vi "Teleop.vi"(10 "Match Info":T1={"Autonomous Elapsed Seconds"=0.0, "TeleOp Elapsed Seconds"=0.0, "Disabled Elapsed Seconds"=0.0, "Visited Autonomous"=FALSE, "Visited TeleOp"=FALSE, "Visited Disabled"=FALSE, "Autonomous Settings"={"Autonomous Style"=enum."Independent", "VI Refnum"=refnum}}, 11 "Call Context":T2) -> ()   [LabVIEW 2019]
doc: "This VI is called for each enabled TeleOp packet received from the DS. It is typically used to read from joysticks and other inputs and update I/O or setpoints for timed control loops. It should complete and return within 20 milliseconds or risk missing DS packets."
uses:
  <vilib>/Rock Robotics/WPI/DriverStation/WPI_DriverStationDerivedRobotMode.ctl
  <vilib>/Rock Robotics/WPI/DriverStation/WPI_DriverStationMatch Info.ctl
  Drive/Implementation/Drive Globals.vi
  <vilib>/Rock Robotics/Network Tables/NT Write Numeric Array.vi
  <vilib>/Rock Robotics/Network Tables/NT Write Boolean Array.vi
panel:
  out "Roller Velocity":dbl
  out "Left LIft Applied Voltage":dbl
  out "Right Drive Velocity":dbl
  out "Left Drive Velocity":dbl
  out "Right LIft Velocity":dbl
  out "Left LIft Velocity":dbl
  out "LeftStopped":bool
  out "RightStopped":bool
  out "Bottom Limit  Pressed":bool
  out "ArmSpeed":dbl
  out "ArmDirection":bool
  out "ArmPosition":dbl
  out "RightDriveSpeed":dbl
  out "RightDriveDirection":bool
  out "RightDriveDistance":dbl
  out "Left Drive Speed":dbl
  out "LeftDriveDirection":bool
  out "LeftDriveDistance":dbl
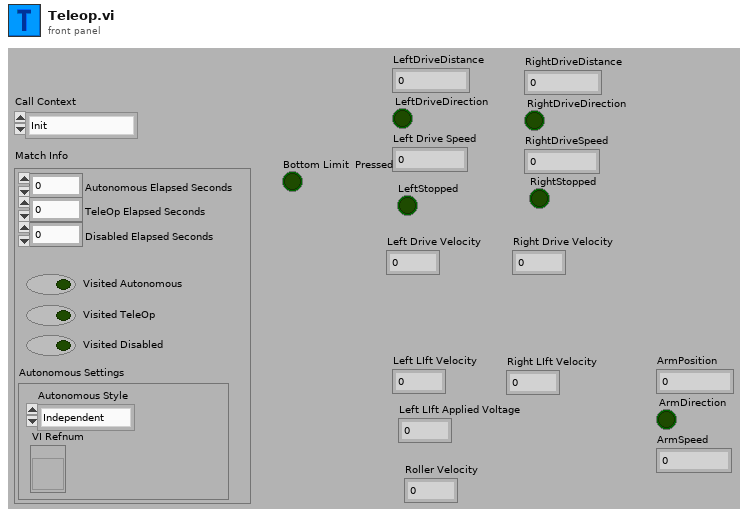
[diagram p1: front panel]
types:
  T1 = typedef "WPI_DriverStationMatch Info.ctl" = cluster{"Autonomous Elapsed Seconds":dbl, "TeleOp Elapsed Seconds":dbl, "Disabled Elapsed Seconds":dbl, "Visited Autonomous":bool, "Visited TeleOp":bool, "Visited Disabled":bool, "Autonomous Settings":cluster{"Autonomous Style":enum16{"Iterative", "Independent"}, "VI Refnum":refnum<vi>}}
  T2 = typedef "WPI_DriverStationDerivedRobotMode.ctl" = enum16{"Init", "Execute", "Stop"}
  T3 = cluster{"Y-Axis":dbl, "Rotation":dbl, "Slider":dbl, "Trigger":bool, "Button 3":bool, "Button 9":bool, "Button 11":bool, "Button 10":bool, "Button 12":bool, "Button 4":bool, "Button 6":bool, "Button 8":bool, "Button 5":bool}
  T4 = typedef "WPI_SwitchDevRef.ctl" = cluster{"DevStatus":errorcluster, "DIO Channel":T5, "CntIndex":T6, "Normally Closed":bool}
  T5 = typedef "FPGA_DIOChannel.ctl" = enum8{"DIO 0", "DIO 1", "DIO 2", "DIO 3", "DIO 4", "DIO 5", "DIO 6", "DIO 7", "DIO 8", "DIO 9", "DIO MXP 0", "DIO MXP 1", "DIO MXP 2", "DIO MXP 3", "DIO MXP 4", "DIO MXP 5", "DIO MXP 6", "DIO MXP 7", "DIO MXP 8", "DIO MXP 9", "DIO MXP 10", "DIO MXP 11", "DIO MXP 12", "DIO MXP 13", "DIO MXP 14", "DIO MXP 15", "SPI Port CS1", "SPI Port CS2", "SPI Port CS3", "SPI Port MISO", "SPI Port MOSI", "Invalid"}
  T6 = typedef "FPGA_CounterCtrSystemIndex.ctl" = enum8{"Ctr 0", "Ctr 1", "Ctr 2", "Ctr 3", "Ctr 4", "Ctr 5", "Ctr 6", "Ctr 7", "Invalid"}
  T7 = typedef "WPI_EncoderDevRef.ctl" = cluster{"DevStatus":errorcluster, "EncoderIndex":T8, "CounterIndex":T6, "DistancePerCount":dbl, "Decoding Type":T9}
  T8 = typedef "FPGA_EncoderIdx.ctl" = enum8{"Enc 0", "Enc 1", "Enc 2", "Enc 3", "Enc 4", "Enc 5", "Enc 6", "Enc 7", "Invalid"}
  T9 = typedef "WPI_EncoderType.ctl" = enum16{"1x", "2x", "4x"}
  T10 = typedef "WPI_JoystickDevRef.ctl" = cluster{"Device":T11}
  T11 = typedef "WPI_JoystickDeviceEnum.ctl" = enum16{"USB 0", "USB 1", "USB 2", "USB 3", "USB 4", "USB 5"}
  T12 = typedef "Command Status Info.ctl" = cluster{"Name":string, "Status":T13, "notifier out":T14}
  T13 = typedef "Completion Status.ctl" = enum16{"Successful", "Aborted", "Incomplete"}
  T14 = typedef "Completion Notifier.ctl" = refnum<notifier>
  T15 = typedef "WPI_MotorControlDeviceRef.ctl" = cluster{"DeviceStatus":errorcluster, "Type":T16, "PWM":cluster{"PWM Channel":T17, "DeadBand":T18}, "CAN":cluster{"Device Number":u8, "SetOutput VI Ref":variant, "GetOutput VI Ref":variant, "Enable VI Ref":variant, "Disable VI Ref":variant, "Data":variant}, "Invert":bool, "DIO PWM":cluster{"PWM \"Enable\" Channel":T17, "DIOChannel":T5, "PWM Rate":dbl}}
  T16 = typedef "WPI_MotorControlType.ctl" = enum16{"PWM", "CAN", "DIO PWM"}
  T17 = typedef "FPGA_DIOPWMChannel.ctl" = enum8{"PWM 0", "PWM 1", "PWM 2", "PWM 3", "PWM 4", "PWM 5", "PWM 6", "PWM 7", "PWM 8", "PWM 9", "PWM MXP 0", "PWM MXP 1", "PWM MXP 2", "PWM MXP 3", "PWM MXP 4", "PWM MXP 5", "PWM MXP 6", "PWM MXP 7", "PWM MXP 8", "PWM MXP 9", "Invalid"}
  T18 = typedef "WPI_PWMDeadband.ctl" = cluster{"Name":string, "maxPositivePwm":i32, "minPositivePwm":i32, "centerPwm":i32, "maxNegativePwm":i32, "minNegativePwm":i32, "angularRange":u16}
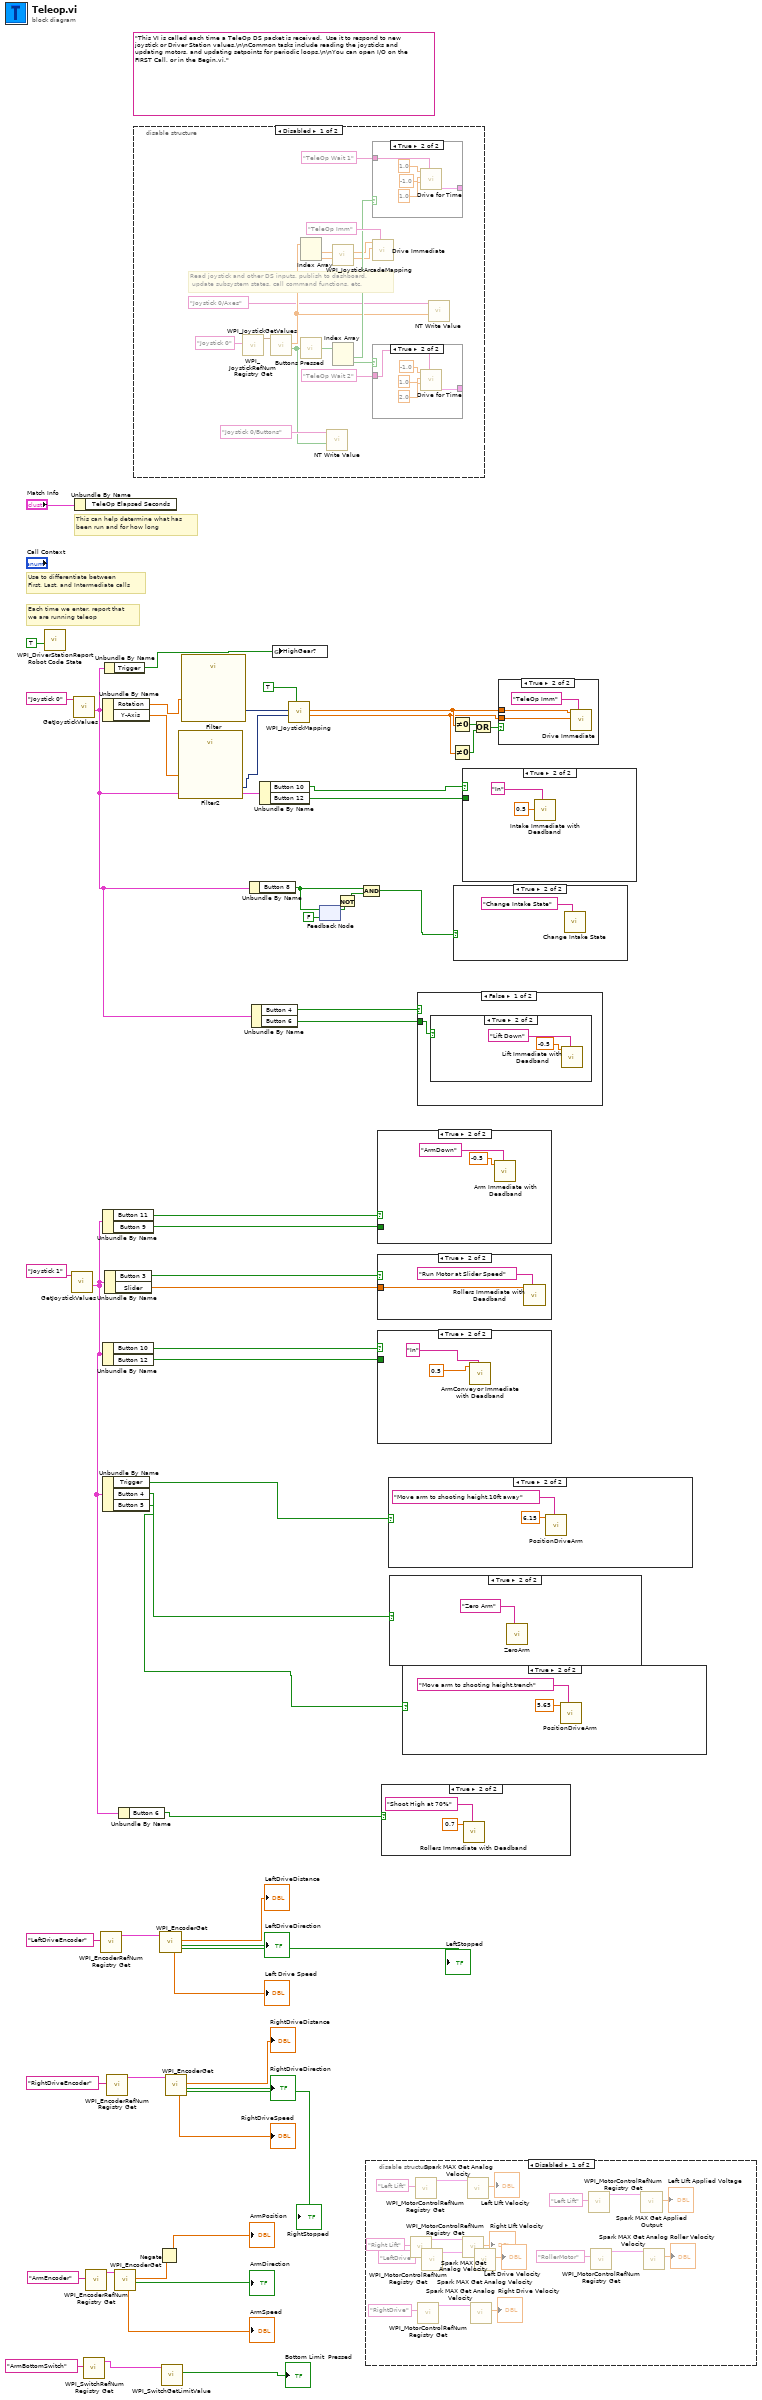
[diagram p0: block diagram]
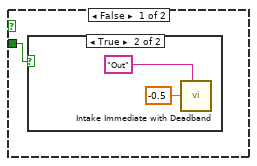
[diagram p8: hidden frame]
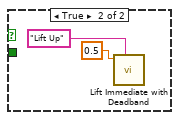
[diagram p11: hidden frame]
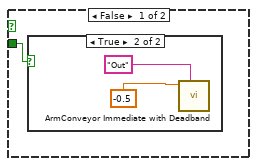
[diagram p12: hidden frame]
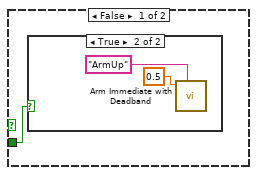
[diagram p14: hidden frame]
diagram:
  (unwired) "This VI is called each time a TeleOp DS packet is received.  Use it to respond to new joystick or Driver Station values.\n\nCommon tasks include reading the joysticks and updating motors, and updating setpoints for periodic loops.\n\nYou can open I/O on the FIRST Call, or in the Begin.vi."
  # "Each time we enter, report that\nwe are running teleop"
  # "Use to differentiate between\nFirst, Last, and Intermediate calls"
  # "This can help determine what has\nbeen run and for how long"
  n1 = call <vilib>:"WPI_DriverStationReport Robot Code State.vi"("TeleOp"=TRUE ("Autonomous")) -> ()  [unwired: 10 in, 1 out]
  n2 = call "GetJoystickValues.vi"("Jockstick Ref"="Joystick 1") -> ("Joystick cluster"=w12:T3)  [unwired: 10 in]
  n3 = call "GetJoystickValues.vi"("Jockstick Ref"="Joystick 0") -> ("Joystick cluster"=w16:T3)  [unwired: 10 in]
  n4 = Unbundle By Name("Match Info") -> ()  [unwired: 1 out]
  n5 = call <vilib>:"WPI_SwitchRefNum Registry Get.vi"("refnum name"="ArmBottomSwitch") -> ("SwitchDevRef"=w20:T4)  [unwired: 9 in, 1 out]
  n6 = call <vilib>:"WPI_EncoderRefNum Registry Get.vi"("refnum name"="ArmEncoder") -> ("EncoderDevRef"=w27:T7)  [unwired: 9 in, 1 out]
  n7 = call <vilib>:"WPI_EncoderRefNum Registry Get.vi"("refnum name"="LeftDriveEncoder") -> ("EncoderDevRef"=w47:T7)  [unwired: 9 in, 1 out]
  n8 = Unbundle By Name(w16) -> ("Rotation"=w9:dbl, "Y-Axis"=w7:dbl)
  n9 = Unbundle By Name(w12) -> ("Button 11"=w32:bool, "Button 9"=w31:bool)
  n10 = Unbundle By Name(w12) -> ("Button 10"=w34:bool, "Button 12"=w33:bool)
  n11 = Unbundle By Name(w12) -> ("Trigger"=w13:bool, "Button 4"=w14:bool, "Button 5"=w6:bool)
  n12 = Unbundle By Name(w16) -> ("Trigger"=w36:bool)
  n13 = Unbundle By Name(w12) -> ("Button 3"=w38:bool, "Slider"=w37:dbl)
  n14 = call <vilib>:"WPI_EncoderRefNum Registry Get.vi"("refnum name"="RightDriveEncoder") -> ("EncoderDevRef"=w42:T7)  [unwired: 9 in, 1 out]
  n15 = call <vilib>:"WPI_EncoderGet.vi"("EncoderDevRef"=w27) -> ("Direction"=→"ArmDirection":bool, "Distance"=w26:dbl, "Rate"=→"ArmSpeed":dbl)  [unwired: 5 in, 3 out]
  n16 = Unbundle By Name(w12) -> ("Button 6"=w11:bool)
  n17 = disable-structure shown="Disabled" {
    frame Disabled {
      # "Read joystick and other DS inputs, publish to dashboard,\n update subsystem states, call command functions, etc."
      n18 = call <vilib>:"WPI_JoystickRefNum Registry Get.vi"("refnum name"="Joystick 0") -> ("JoystickDevRef"=w72:T10)  [unwired: 1 in, 9 out]
      n19 = call <vilib>:"WPI_JoystickGetValues.vi"("JoystickDevRef"=w72) -> ("Buttons"=w60:bool[], "Axes"=w59:dbl[])  [unwired: 6 in, 3 out]
      n20 = Index Array(array=w59) -> (element #1=w63:dbl, element #2=w62:dbl)  [unwired: 2 in]
      n21 = call "Buttons Pressed.vi"("Button Values"=w60) -> ("Button Presses"=w68:bool[])
      n22 = call-poly <vilib>:"NT Write Value.vi"("Boolean Array"=w60, "Name"="Joystick 0/Buttons") -> ()  [unwired: 9 in, 1 out]
      n23 = call <vilib>:"WPI_JoystickArcadeMapping.vi"("Y axis value"=w62, "X axis value"=w63) -> ("Right Motor Value"=w64:dbl, "Left Motor Value"=w65:dbl)  [unwired: 8 in]
      n24 = Index Array(array=w68) -> (element #1=w67:bool, element #2=w66:bool)  [unwired: 2 in]
      n25 = case shown="True" w67 {
        tunnel: [_ w82] -> _
        tunnel: "TeleOp Wait 1" ("Description") -> [_ w81]
        frame False {
        }
        frame True {
          n26 = call "Drive for Time.vi"("Description"=w81, "Seconds"=1.0, "Right Speed"=-1.0, "Left Speed"=1.0) -> ("Command Info Out"=w82:T12)  [unwired: 7 in]
        }
      }
      n27 = call "Drive Immediate.vi"("Description"="TeleOp Imm", "Right Setpoint"=w64, "Left Setpoint"=w65) -> ()  [unwired: 8 in, 1 out]
      n28 = case shown="True" w66 {
        tunnel: [_ w76] -> _
        tunnel: "TeleOp Wait 2" ("Description") -> [_ w75]
        frame False {
        }
        frame True {
          n29 = call "Drive for Time.vi"("Description"=w75, "Seconds"=2.0, "Right Speed"=1.0, "Left Speed"=-1.0) -> ("Command Info Out"=w76:T12)  [unwired: 7 in]
        }
      }
      n30 = call-poly <vilib>:"NT Write Value.vi"("Numeric Array"=w59, "Name"="Joystick 0/Axes") -> ()  [unwired: 9 in, 1 out]
    }
    frame Enabled {
    }
  }
  n31 = Negate(x=w26) -> (-x=→"ArmPosition":dbl)
  n32 = call <vilib>:"WPI_EncoderGet.vi"("EncoderDevRef"=w47) -> ("Direction"=→"LeftDriveDirection":bool, "Distance"=→"LeftDriveDistance":dbl, "Rate"=→"Left Drive Speed":dbl, "Stopped"=→"LeftStopped":bool)  [unwired: 5 in, 2 out]
  n33 = call <vilib>:"WPI_SwitchGetLimitValue.vi"("SwitchDevRef"=w20) -> ("Switch Pressed"=→"Bottom Limit  Pressed":bool)  [unwired: 8 in, 2 out]
  n34 = call <vilib>:"WPI_EncoderGet.vi"("EncoderDevRef"=w42) -> ("Direction"=→"RightDriveDirection":bool, "Distance"=→"RightDriveDistance":dbl, "Rate"=→"RightDriveSpeed":dbl, "Stopped"=→"RightStopped":bool)  [unwired: 5 in, 2 out]
  n35 = call "Filter2"("Signal"=w7) -> ("Filtered Signal"=w8:dynamicdata)  [unwired: 9 in, 1 out]
  n36 = call "Filter"("Signal"=w9) -> ("Filtered Signal"=w10:dynamicdata)  [unwired: 9 in, 1 out]
  n37 = Unbundle By Name(w16) -> ("Button 8"=w4:bool)
  n38 = Unbundle By Name(w16) -> ("Button 4"=w30:bool, "Button 6"=w29:bool)
  n39 = Unbundle By Name(w16) -> ("Button 10"=w22:bool, "Button 12"=w23:bool)
  n40 = global write "Drive Globals.vi" "HighGear?"(w36) -> ()
  n41 = call-poly <vilib>:"WPI_JoystickMapping.vi"("Square Inputs"=TRUE, "Y axis value"=w8, "X axis value"=w10) -> ("Right Motor Value"=w49:dbl, "Left Motor Value"=w50:dbl)  [unwired: 7 in]
  n42 = feedback-in #1(w4) -> ()
  n43 = feedback #1(FALSE ("Button 8")) -> (w5:bool)
  n44 = Not(x=w5) -> (.not. x?=w3:bool)
  n45 = Compound Arithmetic op=AND(w4, w3) -> (w2:bool)
  n46 = disable-structure shown="Disabled" {
    frame Disabled {
      n47 = call <vilib>:"WPI_MotorControlRefNum Registry Get.vi"("refnum name"="Right Lift") -> ("MotorControlDevRef"=w88:T15)  [unwired: 9 in, 1 out]
      n48 = call <vilib>:"WPI_MotorControlRefNum Registry Get.vi"("refnum name"="Left Lift") -> ("MotorControlDevRef"=w86:T15)  [unwired: 9 in, 1 out]
      n49 = call <vilib>:"WPI_MotorControlRefNum Registry Get.vi"("refnum name"="RightDrive") -> ("MotorControlDevRef"=w98:T15)  [unwired: 9 in, 1 out]
      n50 = call <vilib>:"WPI_MotorControlRefNum Registry Get.vi"("refnum name"="LeftDrive") -> ("MotorControlDevRef"=w101:T15)  [unwired: 9 in, 1 out]
      n51 = call <vilib>:"Spark MAX Get Analog Velocity.vi"("MotorControlDevRef in"=w88) -> ("Analog Velocity"=→"Right LIft Velocity":dbl)  [unwired: 7 in, 3 out]
      n52 = call <vilib>:"Spark MAX Get Analog Velocity.vi"("MotorControlDevRef in"=w86) -> ("Analog Velocity"=→"Left LIft Velocity":dbl)  [unwired: 7 in, 3 out]
      n53 = call <vilib>:"Spark MAX Get Analog Velocity.vi"("MotorControlDevRef in"=w98) -> ("Analog Velocity"=→"Right Drive Velocity":dbl)  [unwired: 7 in, 3 out]
      n54 = call <vilib>:"Spark MAX Get Analog Velocity.vi"("MotorControlDevRef in"=w101) -> ("Analog Velocity"=→"Left Drive Velocity":dbl)  [unwired: 7 in, 3 out]
      n55 = call <vilib>:"WPI_MotorControlRefNum Registry Get.vi"("refnum name"="Left Lift") -> ("MotorControlDevRef"=w92:T15)  [unwired: 9 in, 1 out]
      n56 = call <vilib>:"WPI_MotorControlRefNum Registry Get.vi"("refnum name"="RollerMotor") -> ("MotorControlDevRef"=w94:T15)  [unwired: 9 in, 1 out]
      n57 = call <vilib>:"Spark MAX Get Applied Output.vi"("MotorControlDevRef in"=w92) -> ("Applied Output"=→"Left LIft Applied Voltage":dbl)  [unwired: 7 in, 3 out]
      n58 = call <vilib>:"Spark MAX Get Analog Velocity.vi"("MotorControlDevRef in"=w94) -> ("Analog Velocity"=→"Roller Velocity":dbl)  [unwired: 7 in, 3 out]
    }
    frame Enabled {
    }
  }
  n59 = case shown="True" w32 {
    tunnel: w31 -> [w102 _]
    frame False {
      n60 = case shown="True" w102 {
        frame False {
        }
        frame True {
          n61 = call "Arm Immediate with Deadband.vi"("Description"="ArmUp", "Setpoint"=0.5) -> ()  [unwired: 9 in, 1 out]
        }
      }
    }
    frame True {
      n62 = call "Arm Immediate with Deadband.vi"("Description"="ArmDown", "Setpoint"=-0.5) -> ()  [unwired: 9 in, 1 out]
    }
  }
  n63 = case shown="True" w38 {
    tunnel: w37 -> [_ w107]
    frame False {
    }
    frame True {
      n64 = call "Rollers Immediate with Deadband.vi"("Description"="Run Motor at Slider Speed", "Setpoint"=w107) -> ()  [unwired: 9 in, 1 out]
    }
  }
  n65 = case shown="True" w34 {
    tunnel: w33 -> [w109 _]
    frame False {
      n66 = case shown="True" w109 {
        frame False {
        }
        frame True {
          n67 = call "ArmConveyor Immediate with Deadband.vi"("Description"="Out", "Setpoint"=-0.5 ("Intake Setpoint")) -> ()  [unwired: 9 in, 1 out]
        }
      }
    }
    frame True {
      n68 = call "ArmConveyor Immediate with Deadband.vi"("Description"="In", "Setpoint"=0.5 ("Intake Setpoint")) -> ()  [unwired: 9 in, 1 out]
    }
  }
  n69 = case shown="True" w11 {
    frame False {
    }
    frame True {
      n70 = call "Rollers Immediate with Deadband.vi"("Description"="Shoot High at 70%", "Setpoint"=0.7) -> ()  [unwired: 9 in, 1 out]
    }
  }
  n71 = case shown="True" w13 {
    frame False {
    }
    frame True {
      n72 = call "PositionDriveArm.vi"("Description"="Move arm to shooting height,10ft away", "Position"=6.15) -> ()  [unwired: 9 in, 1 out]
    }
  }
  n73 = case shown="True" w14 {
    frame False {
    }
    frame True {
      n74 = call "ZeroArm.vi"("Description"="Zero Arm") -> ()  [unwired: 10 in, 1 out]
    }
  }
  n75 = case shown="True" w6 {
    frame False {
    }
    frame True {
      n76 = call "PositionDriveArm.vi"("Description"="Move arm to shooting height,trench", "Position"=5.65) -> ()  [unwired: 9 in, 1 out]
    }
  }
  n77 = case shown="False" w30 {
    tunnel: w29 -> [w121 _]
    frame False {
      n78 = case shown="True" w121 {
        frame False {
        }
        frame True {
          n79 = call "Lift Immediate with Deadband.vi"("Description"="Lift Down", "Setpoint"=-0.5) -> ()  [unwired: 9 in, 1 out]
        }
      }
    }
    frame True {
      n80 = call "Lift Immediate with Deadband.vi"("Description"="Lift Up", "Setpoint"=0.5) -> ()  [unwired: 9 in, 1 out]
    }
  }
  n81 = Not Equal To 0?(x=w50) -> (x != 0?=w51:bool)
  n82 = Not Equal To 0?(x=w49) -> (x != 0?=w53:bool)
  n83 = case shown="True" w2 {
    frame False {
    }
    frame True {
      n84 = call "Change Intake State.vi"("Description"="Change Intake State") -> ()  [unwired: 10 in, 1 out]
    }
  }
  n85 = case shown="True" w22 {
    tunnel: w23 -> [w127 _]
    frame False {
      n86 = case shown="True" w127 {
        frame False {
        }
        frame True {
          n87 = call "Intake Immediate with Deadband.vi"("Description"="Out", "Intake Setpoint"=-0.5) -> ()  [unwired: 9 in, 1 out]
        }
      }
    }
    frame True {
      n88 = call "Intake Immediate with Deadband.vi"("Description"="In", "Intake Setpoint"=0.5) -> ()  [unwired: 9 in, 1 out]
    }
  }
  n89 = Or(x=w51, y=w53) -> (x .or. y?=w52:bool)
  n90 = case shown="True" w52 {
    tunnel: w50 -> [_ w134]
    tunnel: w49 -> [_ w133]
    frame False {
    }
    frame True {
      n91 = call "Drive Immediate.vi"("Description"="TeleOp Imm", "Right Setpoint"=w133, "Left Setpoint"=w134) -> ()  [unwired: 8 in, 1 out]
    }
  }
